vi "Change Shutter State.vi"(8 "error in":errorcluster, 10 "open":bool, 11 "reference":refnum<k24>) -> (0 "error out":errorcluster, 3 "reference out":refnum<k24>)   [LabVIEW 2020, in "Topas4.lvlib"]
uses:
  Topas4.lvlib
  C:/Windows/SysWOW64/Topas4Lib.dll
  Windows/SysWOW64/Topas4Lib.dll
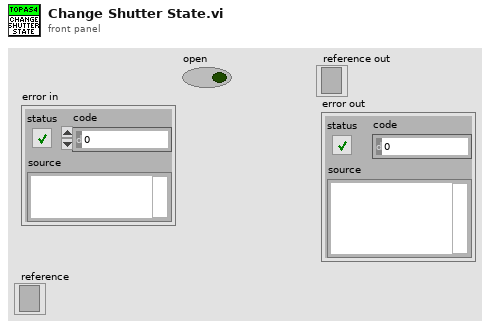
[diagram p1: front panel]
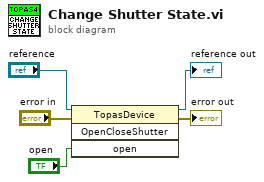
[diagram p0: block diagram]
diagram:
  n1 = invoke class="TopasDevice" method="OpenCloseShutter"(reference="reference", error in="error in", "open"="open") -> (reference out=→"reference out":refnum<k24>, error out=→"error out":errorcluster)  [unwired: 1 in, 2 out]
